vi "Get it done now.vi"(0 "Joystick Command":dbl, 1 "Encoder 0 Distance":dbl, 2 "Encoder 1 Distance":dbl, 7 "Maximum PWM Change":dbl, 9 "Max Following Error":dbl, 11 "error in (no error)":errorcluster) -> (3 "Crash Flag":bool, 6 "Motor 0 Command":dbl, 8 "Motor 1 Command":dbl, 15 "error out":errorcluster)   [LabVIEW 2014]
panel:
  out "Motor 1 Change":dbl
  out "Motor 0 Change":dbl
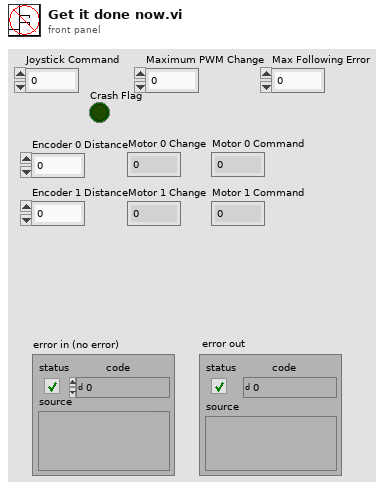
[diagram p1: front panel]
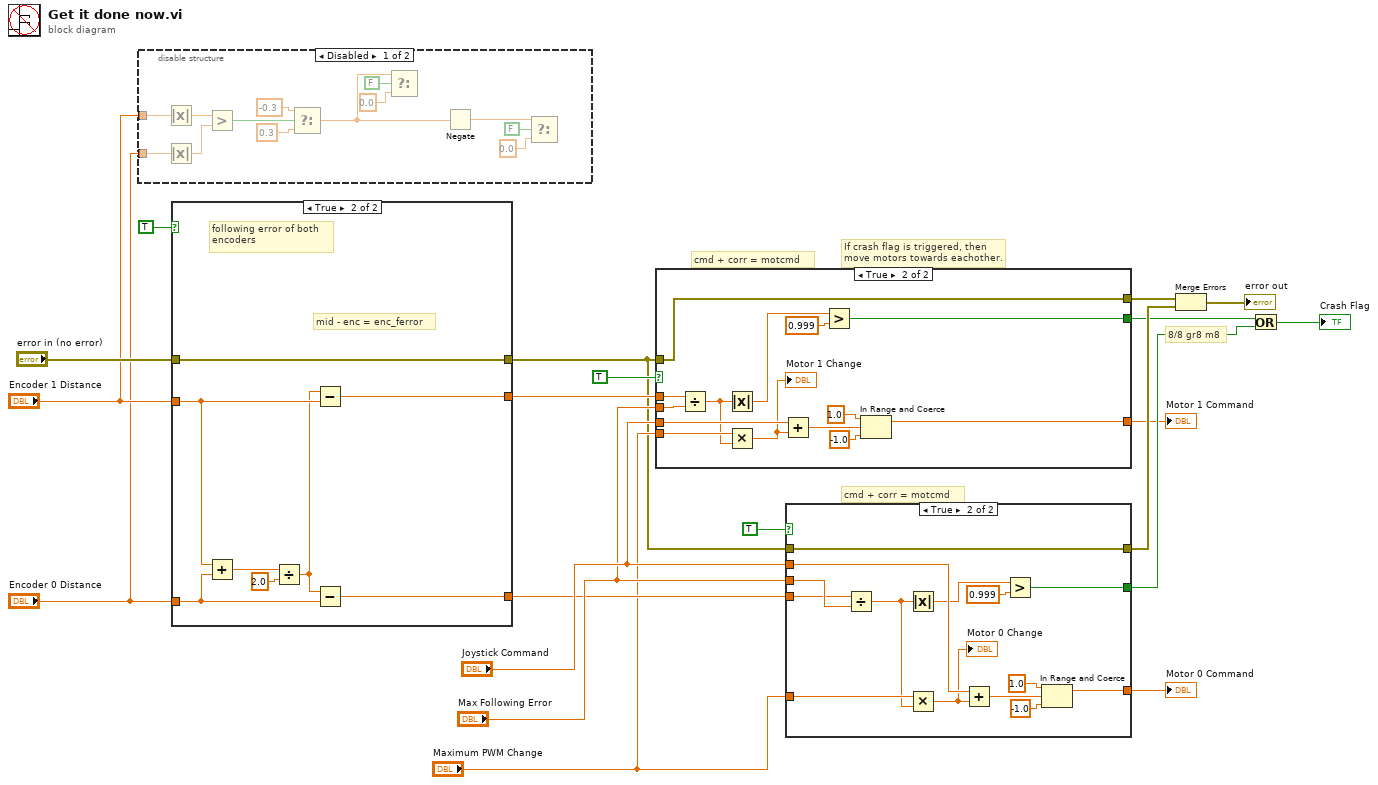
[diagram p0: block diagram]
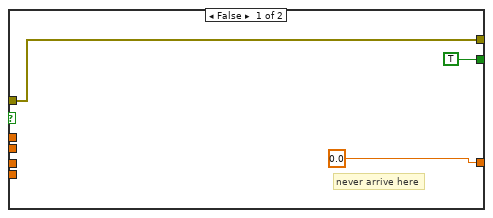
[diagram p3: hidden frame]
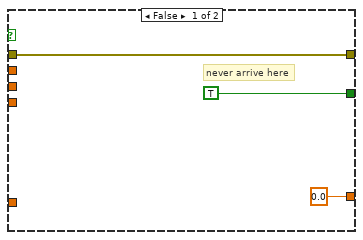
[diagram p4: hidden frame]
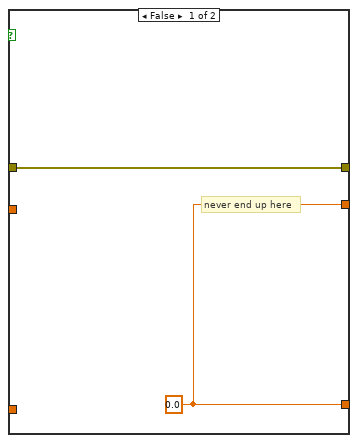
[diagram p5: hidden frame]
diagram:
  # "If crash flag is triggered, then\nmove motors towards eachother."
  # "8/8 gr8 m8"
  # "cmd + corr = motcmd"
  # "cmd + corr = motcmd"
  n1 = disable-structure shown="Disabled" {
    disable-tunnel: "Encoder 1 Distance" -> [w30 _]
    disable-tunnel: "Encoder 0 Distance" -> [w28 _]
    frame Disabled {
      n2 = Absolute Value(x=w30) -> (abs(x)=w29:dbl)
      n3 = Absolute Value(x=w28) -> (abs(x)=w27:dbl)
      n4 = Greater?(x=w29, y=w27) -> (0:w33:bool)
      n5 = Select(t=-0.3, s=w33, f=0.3) -> (s? t:f=w26:dbl)
      n6 = Select(t=w26, s=FALSE, f=0.0) -> ()  [unwired: 1 out]
      n7 = Negate(x=w26) -> (-x=w25:dbl)
      n8 = Select(t=w25, s=FALSE, f=0.0) -> ()  [unwired: 1 out]
    }
    frame Enabled {
    }
  }
  n9 = case shown="True" TRUE {
    tunnel: "Encoder 0 Distance" -> [_ w39]
    tunnel: "Encoder 1 Distance" -> [_ w41]
    tunnel: [w35 w40] -> w15
    tunnel: [w35 w37] -> w14
    tunnel: "error in (no error)" -> [w34 w36]
    tunnel: [w34 w36] -> w11
    frame False {
      w35 = 0.0
      # "never end up here"
    }
    frame True {
      # "mid - enc = enc_ferror"
      # "following error of both\nencoders"
      n10 = Add(x=w41, y=w39) -> (x+y=w42:dbl)
      n11 = Divide(x=w42, y=2.0) -> (x/y=w38:dbl)
      n12 = Subtract(x=w38, y=w41) -> (x-y=w40:dbl)
      n13 = Subtract(x=w38, y=w39) -> (x-y=w37:dbl)
    }
  }
  n14 = case shown="True" TRUE {
    tunnel: w15 -> [_ w57]
    tunnel: "Joystick Command" -> [_ w60]
    tunnel: [0.0 ("f") w47] -> w1
    tunnel: [TRUE w48] -> w7
    tunnel: "Max Following Error" -> [_ w56]
    tunnel: "Maximum PWM Change" -> [_ w55]
    tunnel: w11 -> [w44 w53]
    tunnel: [w44 w53] -> w9
    frame False {
      # "never arrive here"
    }
    frame True {
      n15 = Divide(x=w57, y=w56) -> (x/y=w50:dbl)
      n16 = Absolute Value(x=w50) -> (abs(x)=w49:dbl)
      n17 = Multiply(x=w55, y=w50) -> (x*y=w54:dbl)
      "Motor 1 Change" <- w54
      n18 = Add(x=w60, y=w54) -> (x+y=w58:dbl)
      n19 = Greater?(x=w49, y=0.999) -> (0:w48:bool)
      n20 = In Range and Coerce(upper limit=1.0, x=w58, lower limit=-1.0) -> (coerced(x)=w47:dbl)  [unwired: 1 out]
    }
  }
  "Motor 1 Command" <- w1
  n21 = case shown="True" TRUE {
    tunnel: w14 -> [_ w72]
    tunnel: "Joystick Command" -> [_ w77]
    tunnel: [0.0 ("f") w64] -> w2
    tunnel: [TRUE w66] -> w6
    tunnel: "Max Following Error" -> [_ w73]
    tunnel: "Maximum PWM Change" -> [_ w71]
    tunnel: w11 -> [w61 w69]
    tunnel: [w61 w69] -> w10
    frame False {
      # "never arrive here"
    }
    frame True {
      n22 = Divide(x=w72, y=w73) -> (x/y=w65:dbl)
      n23 = Absolute Value(x=w65) -> (abs(x)=w68:dbl)
      n24 = Multiply(x=w71, y=w65) -> (x*y=w70:dbl)
      "Motor 0 Change" <- w70
      n25 = Add(x=w77, y=w70) -> (x+y=w74:dbl)
      n26 = Greater?(x=w68, y=0.999) -> (0:w66:bool)
      n27 = In Range and Coerce(upper limit=1.0, x=w74, lower limit=-1.0) -> (coerced(x)=w64:dbl)  [unwired: 1 out]
    }
  }
  "Motor 0 Command" <- w2
  n28 = Merge Errors(w9, w10) -> (→"error out":errorcluster)
  n29 = Or(x=w7, y=w6) -> (x .or. y?=→"Crash Flag":bool)
